vi "SERIALsend.vi"(2 "timeout ms":u32=4294967295 format="%.0x", 3 "address string":string, 4 "write buffer":string, 9 "error in":errorcluster) -> (1 "byte count":i32, 6 "error out":errorcluster)   [LabVIEW 2013]
doc: "Sends a string to a message based VXI instrument. In order to communicate with an instrument, you must first open the instrument by running the Open VXI Instrument or running the initialize VI (initialize VIs call the Open VXI Instrument in their block diagram). Use the instrument ID generated by the Open VXI Instrument to address the specific instrument, then set the write mode and enter the string to send. If a write error occurs, error code 1230 is returned. If you fail to open the instrument, error code 1232 is returned."
uses:
  <vilib>/Instr/_visa.llb/VISA Configure Serial Port (Instr).vi
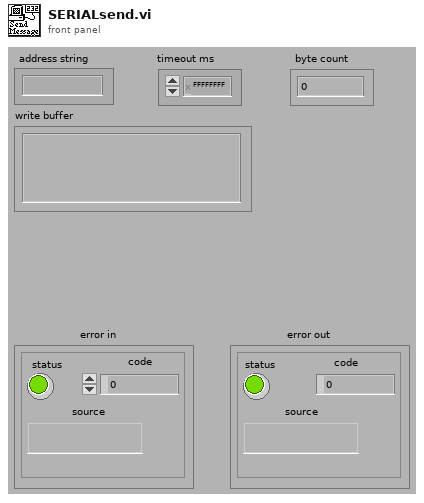
[diagram p1: front panel]
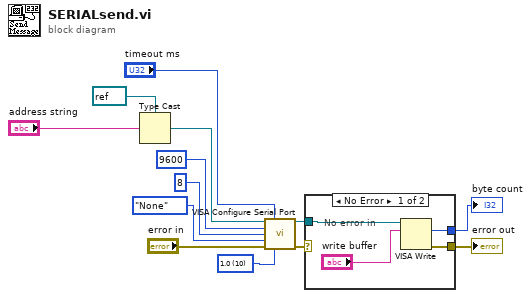
[diagram p0: block diagram]
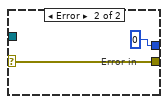
[diagram p2: hidden frame]
diagram:
  w9 = u16 10 items=["1.0"=10, "1.5"=15, "2.0"=20] ("stop bits (10: 1 bit)")
  n1 = Type Cast(type=refnum<visa-resource-name> refnum ("VISA resource name"), x="address string") -> (*(type *) &x=w8:refnum<visa-resource-name>)
  n2 = call-poly "VISA Configure Serial Port"("VISA resource name"=w8, "timeout (10sec)"="timeout ms", "baud rate (9600)"=u32 9600, "data bits (8)"=u16 8, "parity (0:none)"=enum16{"None", "Odd", "Even", "Mark", "Space"}."None", "error in (no error)"="error in", "stop bits (10: 1 bit)"=w9) -> ("VISA resource name out"=w3:refnum<visa-resource-name>, "error out"=w1:errorcluster)  [unwired: 7 in]
  n3 = case shown="No Error" w1 {
    selector: w1 -> [_ w18]
    tunnel: [w16 w18] -> w12
    tunnel: [w15 0] -> w13
    tunnel: w3 -> [w14 _]
    frame No Error {
      # "No error in"
      n4 = VISA Write(VISA resource name=w14, write buffer="write buffer") -> (return count=w15:u32, error out=w16:errorcluster)  [unwired: 1 in, 1 out]
    }
    frame Error {
      # "Error in"
    }
  }
  "error out" <- w12
  "byte count" <- w13
